vi "RunCL - Run All Tests.vi"(11 "CLI Args":string[](array[string])) -> (2 "source":string, 3 "code":i32)   [LabVIEW 2023]
uses:
  <vilib>/addons/_JKI Toolkits/Caraya/classes/Test Report.JUnit/Test Report.JUnit.lvclass
  C:/Program Files/National Instruments/LabVIEW 2023/vi.lib/addons/_JKI Toolkits/Caraya/classes/Test Report/Test Report.lvclass
  <vilib>/addons/_JKI Toolkits/Caraya/classes/Test Runner.Folder/Test Runner.Folder.lvclass
  C:/Program Files/National Instruments/LabVIEW 2023/vi.lib/addons/_JKI Toolkits/Caraya/classes/Test Runner/Test Runner.lvclass
  <userlib>/_OpenG.lib/file/file.llb/Append Path to Root if Relative - Scalar__ogtk.vi
  <userlib>/_OpenG.lib/file/file.llb/File Exists - Scalar__ogtk.vi
  <userlib>/_OpenG.lib/file/file.llb/openg_file.lvlib
  <vilib>/addons/_JKI Toolkits/Caraya/classes/Test Runner/Test Runner.lvclass
panel:
  in  "Show Caraya GUI":bool=TRUE
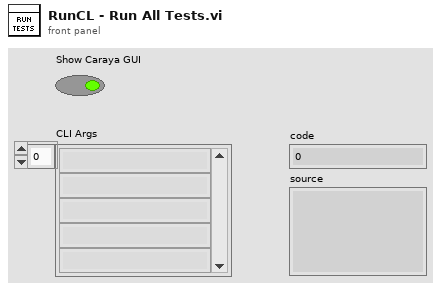
[diagram p1: front panel]
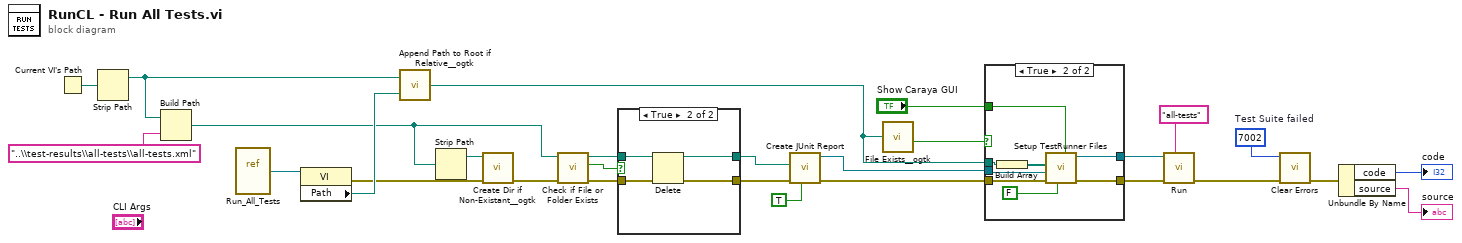
[diagram p0: block diagram]
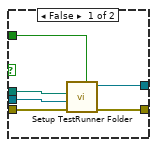
[diagram p2: hidden frame]
diagram:
  w7 = 7002  # Test Suite failed
  n1 = Current VI's Path() -> (path=w27:path)
  n2 = Strip Path(path=w27) -> (stripped path=w8:path)  [unwired: 1 out]
  n3 = Build Path(base path=w8, name or relative path="..\\test-results\\all-tests\\all-tests.xml") -> (appended path=w23:path)
  n4 = vi-ref "Run_All_Tests.vi"() -> (w28:refnum<vi>)
  n5 = property class="VI"(reference=w28) -> (error out=w4:errorcluster, "Path"=w26:path)  [unwired: 1 in, 1 out]
  n6 = call-poly <userlib>:"Append Path to Root if Relative__ogtk.vi"("Absolute or Relative Path"=w26, "Root Path"=w8) -> ("Absolute or Appended Path"=w15:path)
  n7 = Strip Path(path=w23) -> (stripped path=w24:path)  [unwired: 1 out]
  n8 = call <userlib>:"Create Dir if Non-Existant__ogtk.vi"("error in (no error)"=w4, "Directory Path"=w24) -> ("error out"=w11:errorcluster)  [unwired: 7 in, 2 out]
  n9 = call <vilib>:"Check if File or Folder Exists.vi"("error in (no error)"=w11, "path"=w23) -> ("error out"=w10:errorcluster, "file or folder exists?"=w22:bool, "dup path"=w21:path)  [unwired: 7 in]
  n10 = case shown="True" w22 {
    tunnel: w21 -> [w30 w34]
    tunnel: [w30 w33] -> w20
    tunnel: w10 -> [w29 w32]
    tunnel: [w29 w31] -> w9
    frame False {
    }
    frame True {
      n11 = Delete(path (use dialog)=w34, error in=w32) -> (deleted path=w33:path, error out=w31:errorcluster)  [unwired: 3 in, 1 out]
    }
  }
  n12 = call <vilib>:"Create JUnit Report.vi"("Verbose"=TRUE, "error in (no error)"=w9, "Report Path"=w20) -> ("error out"=w12:errorcluster, "Test Report.JUnit out"=w18:refnum<class "Test Report.JUnit.lvclass">)  [unwired: 7 in]
  n13 = call-poly <userlib>:"File Exists__ogtk.vi"("file path"=w15) -> ("exists"=w14:bool)  [unwired: 6 in, 1 out]
  n14 = case shown="True" w14 {
    tunnel: w18 -> [w40 w47]
    tunnel: [w39 w48] -> w17
    tunnel: w15 -> [w38 w45]
    tunnel: [w37 w43] -> w13
    tunnel: w12 -> [w36 w42]
    tunnel: "Show Caraya GUI" -> [w35 w41]
    frame False {
      n15 = call <vilib>:"Setup TestRunner Folder.vi"("Interactive (T)"=w35, "error in (no error)"=w36, "Test Report"=w40, "Directory to search"=w38) -> ("error out"=w37:errorcluster, "Test Runner.Folder out"=w39:refnum<class "Test Runner.Folder.lvclass">)  [unwired: 6 in]
    }
    frame True {
      n16 = Build Array(w45) -> (w44:path[])
      n17 = call <vilib>:"Setup TestRunner Files.vi"("Interactive (T)"=w41, "Inspect Recursively (T)"=FALSE, "error in (no error)"=w42, "Test Report"=w47, "Paths"=w44) -> ("error out"=w43:errorcluster, "Test Runner.Folder out"=w48:refnum<class "Test Runner.Folder.lvclass">)  [unwired: 5 in]
    }
  }
  n18 = call <vilib>:"Run.vi"("Name"="all-tests", "error in (no error)"=w13, "Test Runner in"=w17) -> ("error out"=w6:errorcluster)  [unwired: 6 in, 2 out]
  n19 = call <vilib>:"Clear Errors.vi"("error in (no error)"=w6, "specific error code to clear (0: all)"=w7) -> ("error out"=w3:errorcluster)  [unwired: 4 in, 1 out]
  n20 = Unbundle By Name(w3) -> ("code"=→"code":i32, "source"=→"source":string)
